vi "read_params.vi"(8 "error in (no error)":errorcluster, 11 "SparseCoder in":refnum<class "SparseCoder.lvclass">) -> (0 "error out":errorcluster, 2 "params":T1={"dictionary"=[], "transform_algorithm"="omp", "transform_n_nonzero_coefs"={"transform_n_nonzero_coefs_type"="None", "transform_n_nonzero_coefs_int"=0.0}, "transform_alpha"={"transform_alpha_type"="None", "transform_alpha_float"=0.0}, "split_sign"=FALSE, "n_jobs"=1.0, "positive_code"=FALSE, "transform_max_iter"=1000.0}, 3 "SparseCoder out":refnum<class "SparseCoder.lvclass">)   [LabVIEW 2020, in "SparseCoder.lvclass"]
uses:
  SparseCoder.lvclass
  Controls/sparse_coder_params.ctl
  SparseCoder.lvclass/SparseCoder.ctl
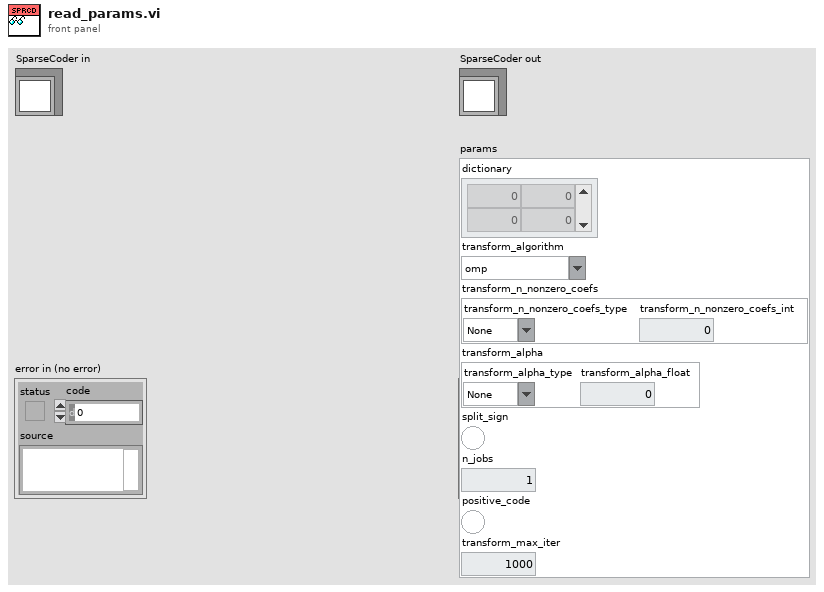
[diagram p1: front panel]
types:
  T1 = typedef "sparse_coder_params.ctl" = cluster{"dictionary":dbl[][], "transform_algorithm":string, "transform_n_nonzero_coefs":cluster{"transform_n_nonzero_coefs_type":string, "transform_n_nonzero_coefs_int":dbl}, "transform_alpha":cluster{"transform_alpha_type":string, "transform_alpha_float":dbl}, "split_sign":bool, "n_jobs":dbl, "positive_code":bool, "transform_max_iter":dbl}
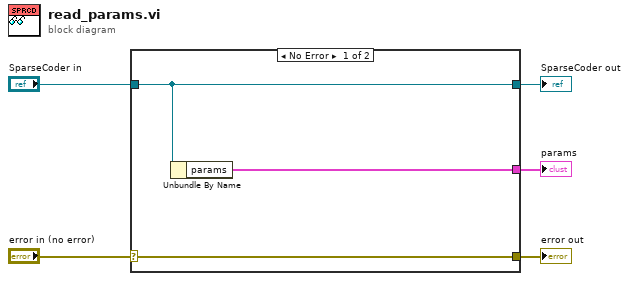
[diagram p0: block diagram]
diagram:
  n1 = case shown="No Error" "error in (no error)" {
    selector: "error in (no error)" -> [w8 w9]
    tunnel: [w8 w9] -> w4
    tunnel: [w7 w10] -> w2
    tunnel: "SparseCoder in" -> [w7 w10]
    tunnel: [w6 _] -> w1
    frame No Error {
      n2 = Unbundle By Name(w7) -> ("params"=w6:T1)
    }
    frame Error {
    }
  }
  "error out" <- w4
  "SparseCoder out" <- w2
  "params" <- w1
